vi "AR-Interlock-monitor-v2.vi"(7 "Action":T2, 8 "error in":errorcluster, 11 "Inlk Com":refnum<visa-resource-name>) -> (0 "error out":errorcluster, 1 "Head F Edge":bool, 2 "Intlk Data Array":T1[](array[typedef]) {"Time Delta (mS)" format="%.3f"}, 3 "Intlk Data":T1 {"Time Delta (mS)" format="%.3f"}, 4 "Raw Output":string)   [LabVIEW 2021]
uses:
  Controls/AR-Interlock-monitor-comands.ctl
  Controls/AR-Interlock-Data.ctl
  <vilib>/Instr/_visa.llb/VISA Flush IO Buffer Mask.ctl
panel:
  out "XY Graph - Dark":cluster{dbl[], i16[]}(graph)
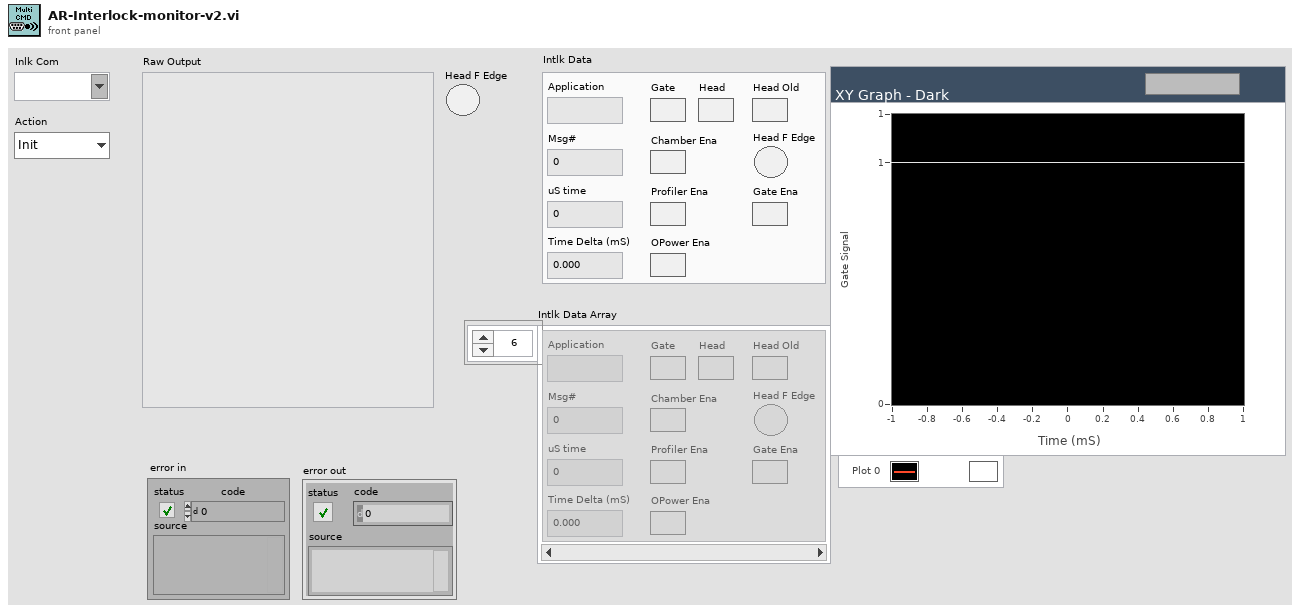
[diagram p1: front panel]
types:
  T1 = typedef "AR-Interlock-Data.ctl" = cluster{"Application":string, "Msg#":i32, "uS time":u32, "Gate":bool, "Head":bool, "Head Old":bool, "Chamber Ena":bool, "Profiler Ena":bool, "OPower Ena":bool, "Gate Ena":bool, "Time Delta (mS)":dbl, "Head F Edge":bool}
  T2 = typedef "AR-Interlock-monitor-comands.ctl" = enum16{"Init", "Request", "Poll Serial", "Close", "Clear Data"}
  T3 = cluster{"Baud Rate":u32, "Parity":u16, "Data Bits":u16, "Serial Settings:Serial Flow Control":u16, "Serial Port":u16, "Serial Settings:Serial Stop Bits":u16}
  T4 = typedef "VISA Flush IO Buffer Mask.ctl" = u16
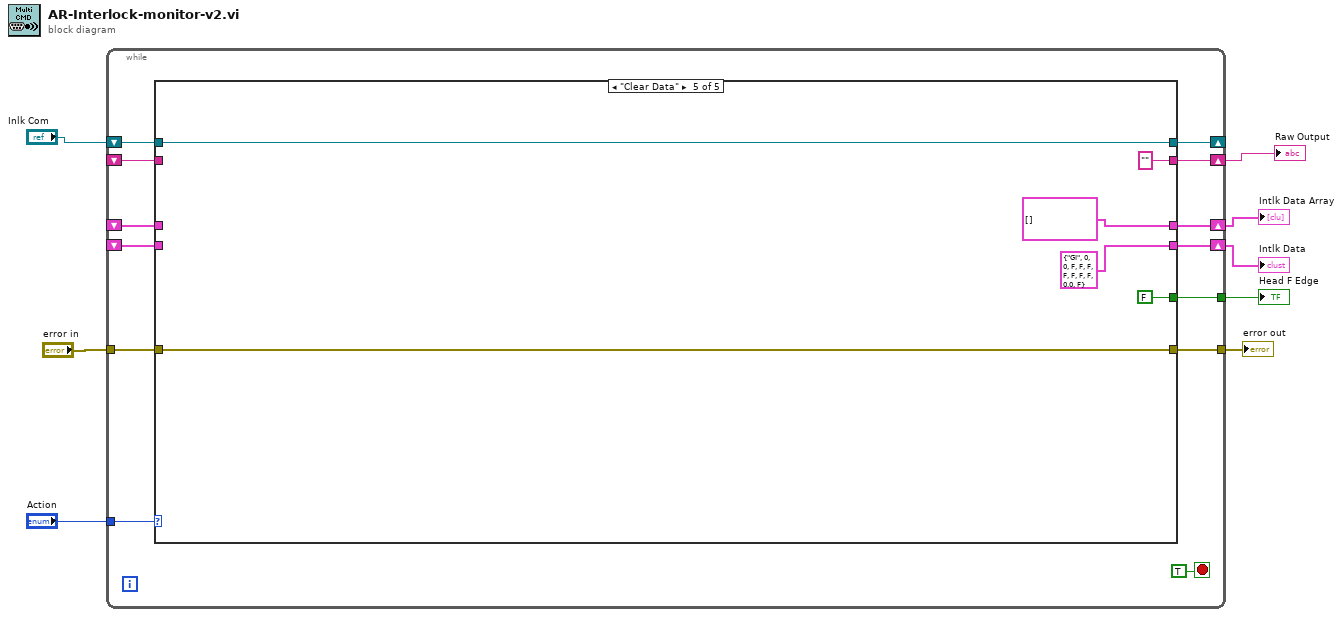
[diagram p0: block diagram]
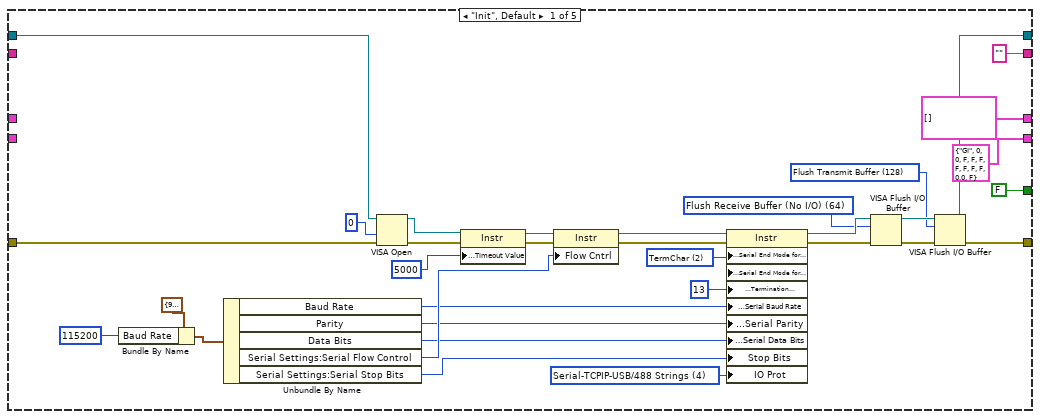
[diagram p2: hidden frame]
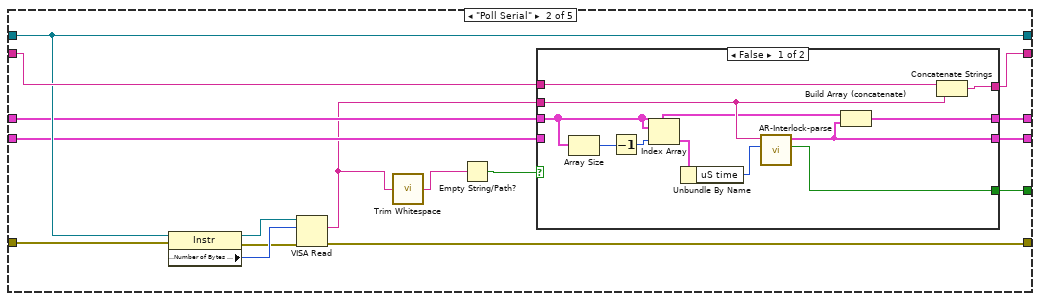
[diagram p3: hidden frame]
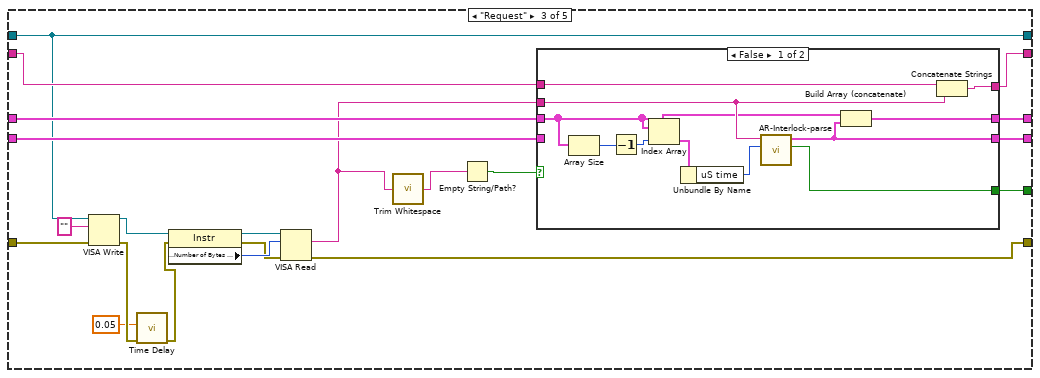
[diagram p5: hidden frame]
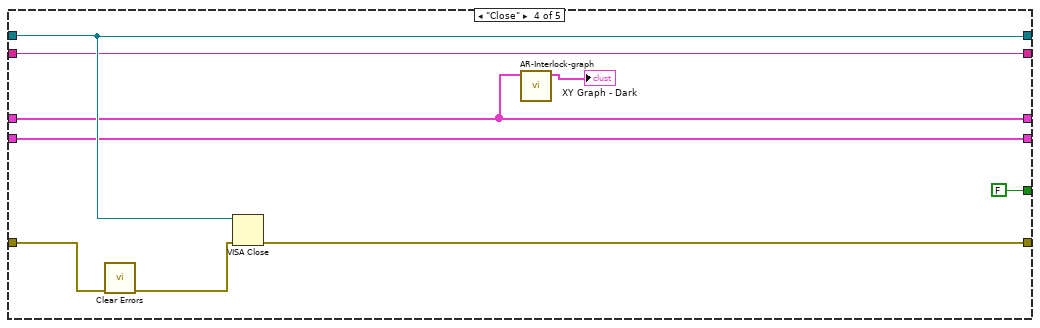
[diagram p7: hidden frame]
diagram:
  n1 = while {
    tunnel: "Action" -> [w20]
    tunnel: "error in" -> [w19]
    tunnel: [w18] -> w5
    shift-right: [w17] -> _
    shift-left: "Inlk Com" -> [w15]
    shift-right: [w16] -> w6
    shift-left: _ -> [w14]
    shift-right: [w12] -> w4
    shift-left: _ -> [w11]
    shift-right: [w13] -> w3
    shift-left: _ -> [w10]
    tunnel: [w9] -> w2
    stop <- TRUE stop-if-true
    n2 = case shown="\"Clear Data\"" w20 {
      tunnel: w19 -> [w29 w66 w91 w128 w129]
      tunnel: [w28 w67 w102 w126 w129] -> w18
      tunnel: [w27 w62 w90 w125 w134] -> w17
      tunnel: ["" ("read buffer") w64 w100 w124 "" ("read buffer")] -> w16
      tunnel: w15 -> [w22 w62 w90 w125 w134]
      tunnel: w14 -> [_ w63 w99 w124 _]
      tunnel: [T1 {"Application"="GI", "Msg#"=0, "uS time"=0, "Gate"=FALSE, "Head"=FALSE, "Head Old"=FALSE, "Chamber Ena"=FALSE, "Profiler Ena"=FALSE, "OPower Ena"=FALSE, "Gate Ena"=FALSE, "Time Delta (mS)"=0.0, "Head F Edge"=FALSE} ("Intlk Data") w61 w98 w123 T1 {"Application"="GI", "Msg#"=0, "uS time"=0, "Gate"=FALSE, "Head"=FALSE, "Head Old"=FALSE, "Chamber Ena"=FALSE, "Profiler Ena"=FALSE, "OPower Ena"=FALSE, "Gate Ena"=FALSE, "Time Delta (mS)"=0.0, "Head F Edge"=FALSE} ("Intlk Data")] -> w13
      tunnel: [T1[] [] w60 w97 w121 T1[] []] -> w12
      tunnel: w11 -> [_ w59 w96 w121 _]
      tunnel: w10 -> [_ w58 w95 w123 _]
      tunnel: [FALSE ("Head F Edge") w55 w92 FALSE ("Head F Edge") FALSE ("Head F Edge")] -> w9
      frame "Init", Default {
        w31 = T4 128 items=["Flush Receive Buffer"=16, "Write Transmit Buffer to Device"=32, "Flush Receive Buffer (No I/O)"=64, "Flush Transmit Buffer"=128] ("Mask")
        w34 = T4 64 items=["Flush Receive Buffer"=16, "Write Transmit Buffer to Device"=32, "Flush Receive Buffer (No I/O)"=64, "Flush Transmit Buffer"=128] ("Mask")
        w45 = u16 2 items=["None", "LastBit", "TermChar"] ("Serial Settings:Serial End Mode for Reads")
        w41 = u16 4 items=["Normal"=1, "VXI/FDC"=2, "GPIB/HS488"=3, "Serial-TCPIP-USB/488 Strings"=4, "USBTMC/Vendor-Specific"=5] ("Message Based Settings:IO Protocol")
        n3 = Bundle By Name(cluster=T3 {"Baud Rate"=9600, "Parity"=0, "Data Bits"=8, "Serial Settings:Serial Flow Control"=0, "Serial Port"=6, "Serial Settings:Serial Stop Bits"=10} ("Serial Configuration"), "Baud Rate"=u32 115200) -> (w37:T3)
        n4 = Unbundle By Name(w37) -> ("Baud Rate"=w44:u32, "Parity"=w43:u16, "Data Bits"=w42:u16, "Serial Settings:Serial Flow Control"=w48:u16, "Serial Settings:Serial Stop Bits"=w40:u16)
        n5 = VISA Open(access mode=u32 0, error in (no error)=w29, VISA resource name=w22) -> (VISA resource name=w52:refnum<visa-resource-name>, error out=w53:errorcluster)  [unwired: 2 in]
        n6 = property on="Property Node" class="Instr"(reference=w52, error in=w53, "General Settings:Timeout Value"=u32 5000 ("Timeout [ms]")) -> (reference out=w50:refnum<visa-resource-name>, error out=w49:errorcluster)
        n7 = property on="Property Node" class="Instr"(reference=w50, error in=w49, "Flow Cntrl"=w48) -> (reference out=w47:refnum<visa-resource-name>, error out=w46:errorcluster)
        n8 = property on="Property Node" class="Instr"(reference=w47, error in=w46, "Serial Settings:Serial End Mode for Reads"=w45, "Serial Settings:Serial End Mode for Writes"=w45, "Message Based Settings:Termination Character"=u8 13, "Serial Settings:Serial Baud Rate"=w44, "Serial Settings:Serial Parity"=w43, "Serial Settings:Serial Data Bits"=w42, "Stop Bits"=w40, "IO Prot"=w41) -> (reference out=w36:refnum<visa-resource-name>, error out=w35:errorcluster)
        n9 = VISA Flush I/O Buffer(VISA resource name=w36, mask (16)=w34, error in (no error)=w35) -> (VISA resource name out=w33:refnum<visa-resource-name>, error out=w32:errorcluster)
        n10 = VISA Flush I/O Buffer(VISA resource name=w33, mask (16)=w31, error in (no error)=w32) -> (VISA resource name out=w27:refnum<visa-resource-name>, error out=w28:errorcluster)
      }
      frame "Poll Serial" {
        n11 = property class="Instr"(reference=w62, error in=w66) -> (reference out=w70:refnum<visa-resource-name>, error out=w68:errorcluster, "Serial Settings:Number of Bytes at Serial Port"=w69:u32)
        n12 = VISA Read(VISA resource name=w70, byte count=w69, error in (no error)=w68) -> (read buffer=w57:string, error out=w67:errorcluster)  [unwired: 2 out]
        n13 = call <vilib>:"Trim Whitespace.vi"("string"=w57) -> ("trimmed string"=w56:string)  [unwired: 1 in]
        n14 = Empty String/Path?(string/path=w56) -> (empty?=w65:bool)
        n15 = case shown="False" w65 {
          tunnel: w57 -> [w79 _]
          tunnel: w63 -> [w81 w84]
          tunnel: [w80 w84] -> w64
          tunnel: [w78 w82] -> w61
          tunnel: [w77 w83] -> w60
          tunnel: w59 -> [w74 w83]
          tunnel: w58 -> [_ w82]
          tunnel: [w71 _] -> w55
          frame False {
            n16 = Array Size(array=w74) -> (size(s)=w76:i32)
            n17 = Decrement(x=w76) -> (x-1=w75:i32)
            n18 = Index Array(array=w74, index=w75) -> (element=w73:T1)
            n19 = Unbundle By Name(w73) -> ("uS time"=w72:u32)
            n20 = call "AR-Interlock-parse.vi"("Perv uS time"=w72, "Str in"=w79) -> ("Head F Edge"=w71:bool, "Intlk Data"=w78:T1)  [unwired: 6 in, 2 out]
            n21 = Build Array (concatenate)(w74, w78) -> (w77:T1[])
            n22 = Concatenate Strings(w81, w79) -> (w80:string)
          }
          frame True {
          }
        }
      }
      frame "Request" {
        n23 = VISA Write(VISA resource name=w90, write buffer="", error in (no error)=w91) -> (VISA resource name out=w89:refnum<visa-resource-name>, error out=w87:errorcluster)  [unwired: 1 out]
        n24 = call "Time Delay"("error in (no error)"=w87, "Delay Time (s)"=0.05) -> ("error out"=w86:errorcluster)  [unwired: 9 in]
        n25 = property class="Instr"(reference=w89, error in=w86) -> (reference out=w105:refnum<visa-resource-name>, error out=w103:errorcluster, "Serial Settings:Number of Bytes at Serial Port"=w104:u32)
        n26 = VISA Read(VISA resource name=w105, byte count=w104, error in (no error)=w103) -> (read buffer=w94:string, error out=w102:errorcluster)  [unwired: 2 out]
        n27 = call <vilib>:"Trim Whitespace.vi"("string"=w94) -> ("trimmed string"=w93:string)  [unwired: 1 in]
        n28 = Empty String/Path?(string/path=w93) -> (empty?=w101:bool)
        n29 = case shown="False" w101 {
          tunnel: w94 -> [w114 _]
          tunnel: w99 -> [w116 w119]
          tunnel: [w115 w119] -> w100
          tunnel: [w113 w117] -> w98
          tunnel: [w112 w118] -> w97
          tunnel: w96 -> [w109 w118]
          tunnel: w95 -> [_ w117]
          tunnel: [w106 _] -> w92
          frame False {
            n30 = Array Size(array=w109) -> (size(s)=w111:i32)
            n31 = Decrement(x=w111) -> (x-1=w110:i32)
            n32 = Index Array(array=w109, index=w110) -> (element=w108:T1)
            n33 = Unbundle By Name(w108) -> ("uS time"=w107:u32)
            n34 = call "AR-Interlock-parse.vi"("Perv uS time"=w107, "Str in"=w114) -> ("Head F Edge"=w106:bool, "Intlk Data"=w113:T1)  [unwired: 6 in, 2 out]
            n35 = Build Array (concatenate)(w109, w113) -> (w112:T1[])
            n36 = Concatenate Strings(w116, w114) -> (w115:string)
          }
          frame True {
          }
        }
      }
      frame "Close" {
        n37 = call <vilib>:"Clear Errors.vi"("error in (no error)"=w128) -> ("error out"=w127:errorcluster)  [unwired: 5 in, 1 out]
        n38 = VISA Close(VISA resource name=w125, error in (no error)=w127) -> (error out=w126:errorcluster)
        n39 = call "AR-Interlock-graph.vi"("Intlk Data Array"=w121) -> ("Gate"=→"XY Graph - Dark":cluster{dbl[], i16[]})  [unwired: 8 in, 2 out]
      }
      frame "Clear Data" {
      }
    }
  }
  "Raw Output" <- w6
  "error out" <- w5
  "Intlk Data Array" <- w4
  "Intlk Data" <- w3
  "Head F Edge" <- w2
